vi "Enqueue Single Msg.vi"(8 "error in":errorcluster, 9 "enable (T)":bool=TRUE, 11 "queue/message":string) -> (0 "error out":errorcluster)   [LabVIEW 2021]
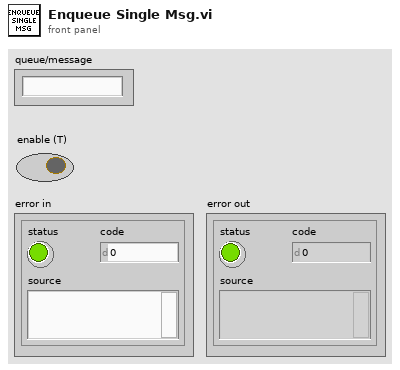
[diagram p1: front panel]
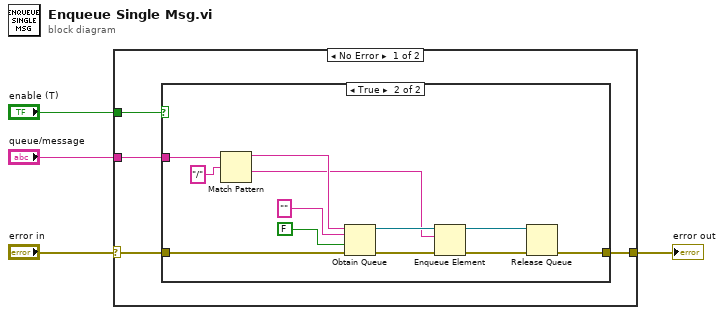
[diagram p0: block diagram]
diagram:
  n1 = case shown="No Error" "error in" {
    selector: "error in" -> [w6 w22]
    tunnel: "enable (T)" -> [w8 _]
    tunnel: "queue/message" -> [w7 _]
    tunnel: [w5 w22] -> w1
    frame No Error {
      n2 = case shown="True" w8 {
        tunnel: w7 -> [_ w21]
        tunnel: w6 -> [w9 w11]
        tunnel: [w9 w13] -> w5
        frame False {
        }
        frame True {
          n3 = Match Pattern(string=w21, regular expression="/") -> (before substring=w19:string, after substring=w14:string)  [unwired: 1 in, 2 out]
          n4 = Obtain Queue(name (unnamed)=w19, element data type="", create if not found? (T)=FALSE, error in (no error)=w11) -> (queue out=w16:refnum<queue>, error out=w10:errorcluster)  [unwired: 1 in, 1 out]
          n5 = Enqueue Element(queue=w16, element=w14, error in (no error)=w10) -> (queue out=w15:refnum<queue>, error out=w12:errorcluster)  [unwired: 1 in, 1 out]
          n6 = Release Queue(queue=w15, error in (no error)=w12) -> (error out=w13:errorcluster)  [unwired: 1 in, 2 out]
        }
      }
    }
    frame Error {
    }
  }
  "error out" <- w1
